vi "ACT_Loop.vi"() -> ()   [LabVIEW 2023, in "Angler_ACT.lvlib"]
uses:
  Angler_ACT.lvlib
  Cluster_CMD_ACT_Data.ctl
  ENUM_Input Mode.ctl
  Type Defs/Cluster_Angler_Angle to Position.ctl
  ENUM_ACT_State.ctl
  <vilib>/Rock Robotics/WPI/MotorControl/WPI_MotorControlDeviceRef.ctl
  <vilib>/Rock Robotics/WPI/MotorControl/WPI_MotorControlType.ctl
  <vilib>/Rock Robotics/SystemInterfaces/DIO/FPGA_DIOPWMChannel.ctl
  <vilib>/Rock Robotics/WPI/PWM/WPI_PWMDeadband.ctl
  <vilib>/Rock Robotics/SystemInterfaces/DIO/FPGA_DIOChannel.ctl
  <vilib>/Rock Robotics/WPI/ThirdParty/Phoenix-LabVIEW/Motor Controller/Controls/CTRE_Phoenix_MotorControl_NeutralMode.ctl
  <vilib>/Rock Robotics/WPI/ThirdParty/Phoenix-LabVIEW/Motor Controller/Controls/CTRE_Phoenix_MotorControl_ControlMode.ctl
  ENUM_ACT_Action.ctl
  RoboRIO Utilities/Global_STOP.vi
  Global_CMD_ACT_Data In.vi
  <vilib>/Rock Robotics/WPI/ThirdParty/Phoenix-LabVIEW/Motor Controller/Get/CTRE_Phoenix_MotorController_GetSelectedSensorData.vi
  <vilib>/Rock Robotics/WPI/ThirdParty/Phoenix-LabVIEW/Motor Controller/Get/CTRE_Phoenix_MotorController_GetClosedLoopData.vi
  Global_ACT_Data Out.vi
panel:
  in  "Max Speed":dbl=0.5
  out "Position Error":i32
  out "Current Angle":dbl
  in  "Angle vs Positon Table":T1[](array[typedef])=[{"Angle"=11.5, "Count"=100}, {"Angle"=15.0, "Count"=156}, {"Angle"=20.0, "Count"=231}, {"Angle"=25.0, "Count"=308}, {"Angle"=30.0, "Count"=386}, {"Angle"=35.0, "Count"=466}, {"Angle"=36.5, "Count"=480}]
  out "Target Unit Positon":dbl
  out "Input Angler Data":T2
  out "Sensor Positon":i32
  out "Cycle Time (S)":dbl format="%.3g"
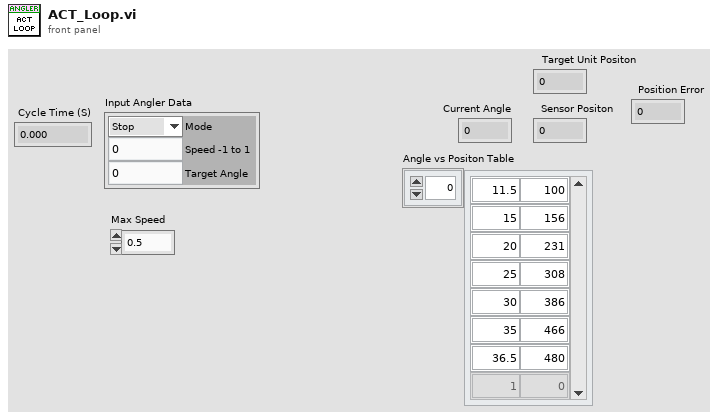
[diagram p1: front panel]
types:
  T1 = typedef "Cluster_Angler_Angle to Position.ctl" = cluster{"Angle":dbl, "Count":i32}
  T2 = typedef "Angler_ACT.lvlib/Cluster_CMD_ACT_Data.ctl" = cluster{"Mode":T3, "Speed -1 to 1":dbl, "Target Angle":dbl}
  T3 = typedef "Angler_ACT.lvlib/ENUM_Input Mode.ctl" = enum16{"Stop", "Speed", "Angle"}
  T4 = typedef "CTRE_Phoenix_MotorControl_ControlMode.ctl" = u16
  T5 = typedef "CTRE_Phoenix_MotorControl_NeutralMode.ctl" = enum8{"EEPROMSetting", "Override to Coast", "Override to Brake"}
  T6 = typedef "WPI_MotorControlDeviceRef.ctl" = cluster{"DeviceStatus":errorcluster, "Type":T7, "PWM":cluster{"PWM Channel":T8, "DeadBand":T9}, "CAN":cluster{"Device Number":u8, "SetOutput VI Ref":variant, "GetOutput VI Ref":variant, "Enable VI Ref":variant, "Disable VI Ref":variant, "Data":variant}, "Invert":bool, "DIO PWM":cluster{"PWM \"Enable\" Channel":T8, "DIOChannel":T10, "PWM Rate":dbl}}
  T7 = typedef "WPI_MotorControlType.ctl" = enum16{"PWM", "CAN", "DIO PWM"}
  T8 = typedef "FPGA_DIOPWMChannel.ctl" = enum8{"PWM 0", "PWM 1", "PWM 2", "PWM 3", "PWM 4", "PWM 5", "PWM 6", "PWM 7", "PWM 8", "PWM 9", "PWM MXP 0", "PWM MXP 1", "PWM MXP 2", "PWM MXP 3", "PWM MXP 4", "PWM MXP 5", "PWM MXP 6", "PWM MXP 7", "PWM MXP 8", "PWM MXP 9", "Invalid"}
  T9 = typedef "WPI_PWMDeadband.ctl" = cluster{"Name":string, "maxPositivePwm":i32, "minPositivePwm":i32, "centerPwm":i32, "maxNegativePwm":i32, "minNegativePwm":i32, "angularRange":u16}
  T10 = typedef "FPGA_DIOChannel.ctl" = enum8{"DIO 0", "DIO 1", "DIO 2", "DIO 3", "DIO 4", "DIO 5", "DIO 6", "DIO 7", "DIO 8", "DIO 9", "DIO MXP 0", "DIO MXP 1", "DIO MXP 2", "DIO MXP 3", "DIO MXP 4", "DIO MXP 5", "DIO MXP 6", "DIO MXP 7", "DIO MXP 8", "DIO MXP 9", "DIO MXP 10", "DIO MXP 11", "DIO MXP 12", "DIO MXP 13", "DIO MXP 14", "DIO MXP 15", "SPI Port CS1", "SPI Port CS2", "SPI Port CS3", "SPI Port MISO", "SPI Port MOSI", "Invalid"}
  T11 = typedef "Angler_ACT.lvlib/ENUM_ACT_State.ctl" = enum16{"Starting", "Stopping", "Ending", "Setting Speed", "Going to Angle"}
  T12 = typedef "Angler_ACT.lvlib/ENUM_ACT_Action.ctl" = enum16{"No Action", "Reset Time", "Reset All", "Stop", "Set Speed", "Set Target Position", "Calculate Target Position from Angle", "Set Soft Limits", "Set Min Motor Value", "Set Current Limit"}
  T13 = cluster{"Angler Motor Ref":T6, "State":T11, "Previous State":T11, "Current Time":timestamp, "Previous Time":timestamp, "Start Time":timestamp, "Target Time (ms)":u32, "Cycle Time(S)":dbl, "ACT Input":T2, "Target Unit Positon":dbl, "Current Angle":dbl, "Sensor Unit Position":i32, "Lower Soft Limit":bool, "Upper Soft Limit":bool, "Sensor Velocity":i32, "Control Mode":T4, "Motor Value":dbl, "Angle Array":dbl[], "Position Array":i32[], "Speed Limit":dbl, "Position Error":i32, "Min Motor Output":dbl, "Max Current":i32}
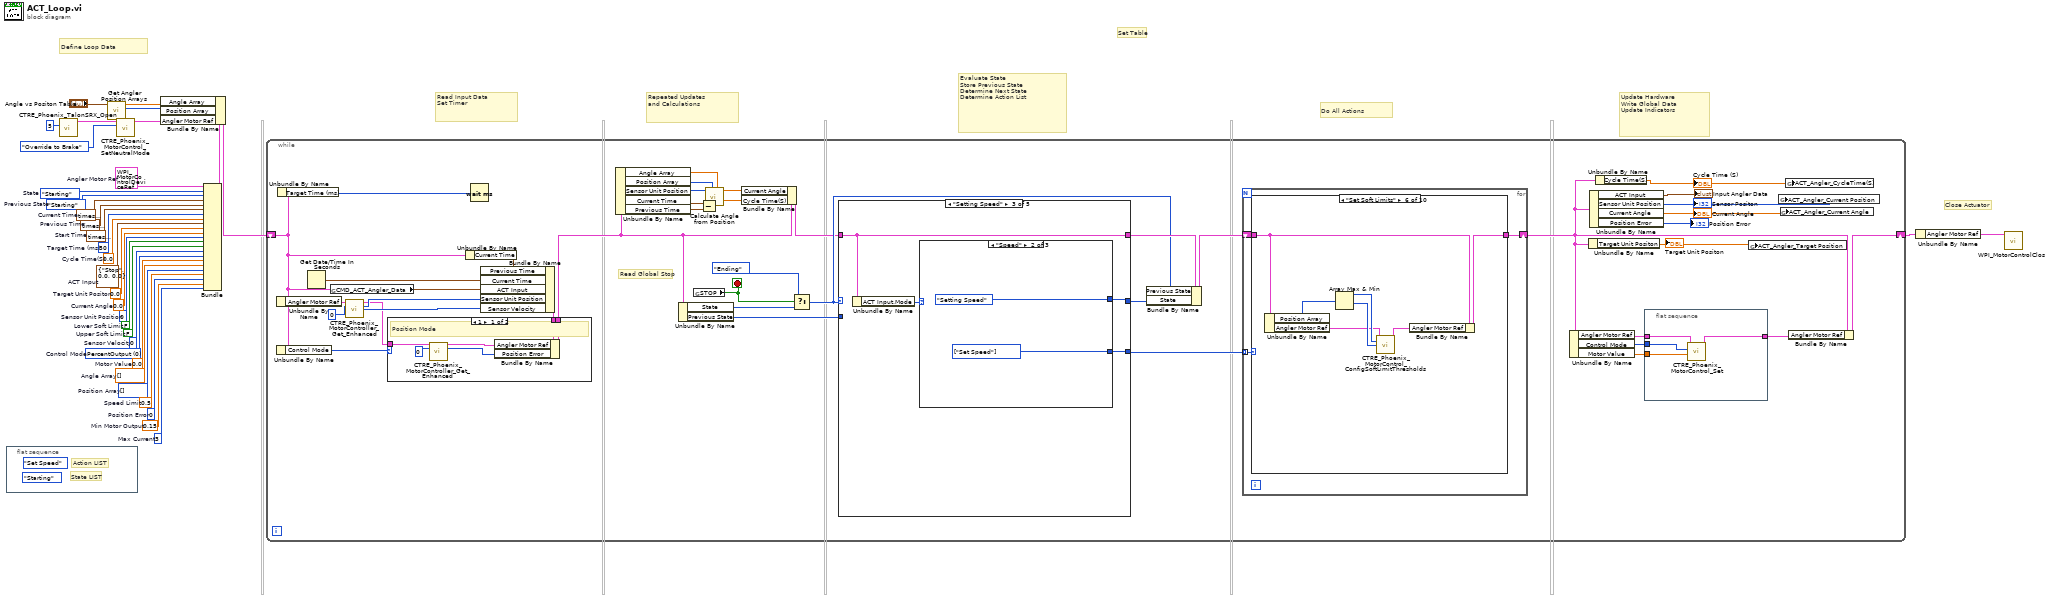
[diagram p0: block diagram]
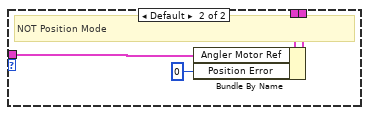
[diagram p2: hidden frame]
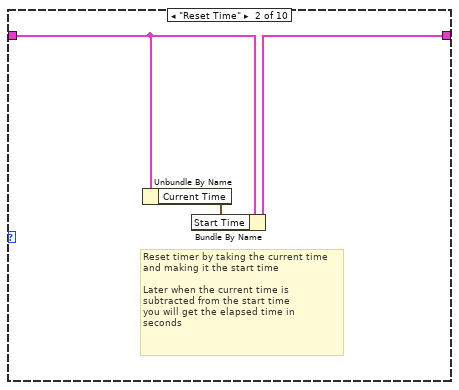
[diagram p4: hidden frame]
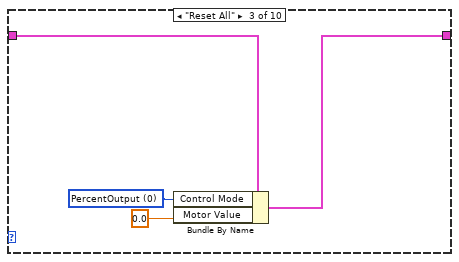
[diagram p5: hidden frame]
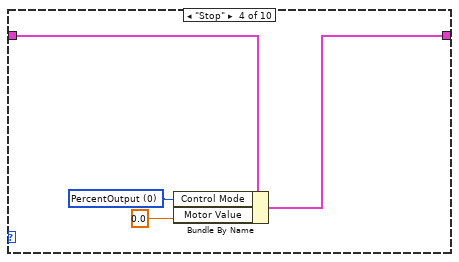
[diagram p6: hidden frame]
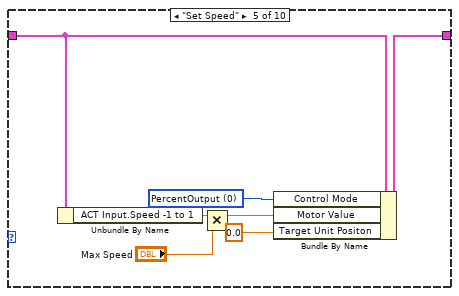
[diagram p7: hidden frame]
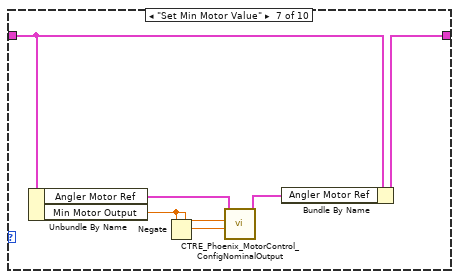
[diagram p8: hidden frame]
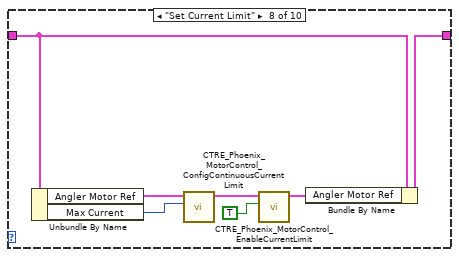
[diagram p9: hidden frame]
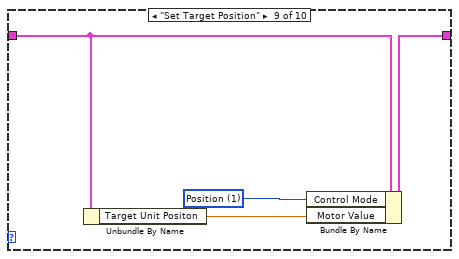
[diagram p10: hidden frame]
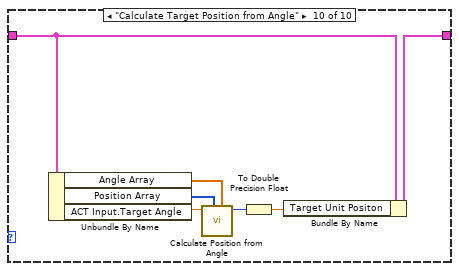
[diagram p11: hidden frame]
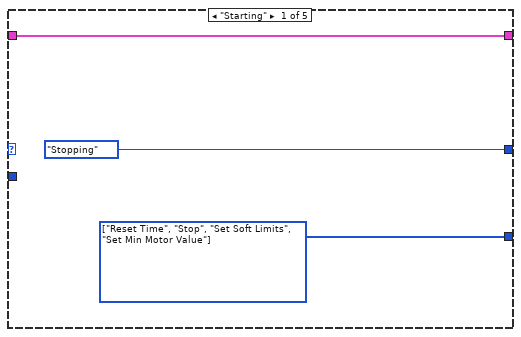
[diagram p12: hidden frame]
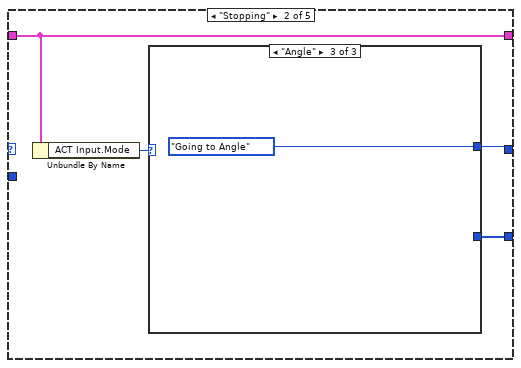
[diagram p13: hidden frame]
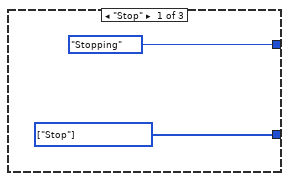
[diagram p14: hidden frame]
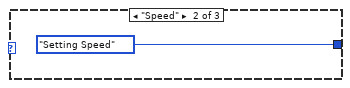
[diagram p15: hidden frame]
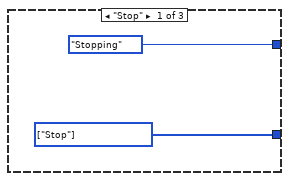
[diagram p16: hidden frame]
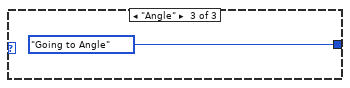
[diagram p17: hidden frame]
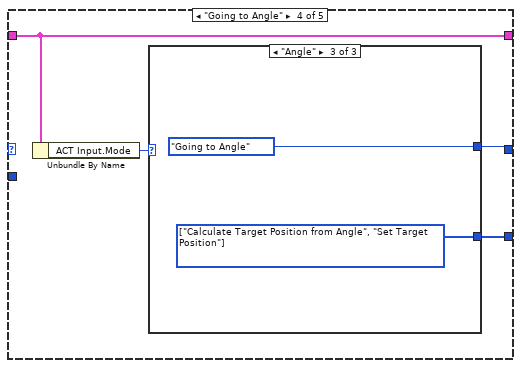
[diagram p18: hidden frame]
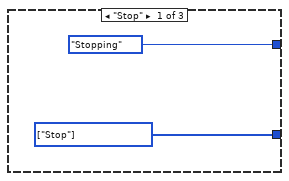
[diagram p19: hidden frame]
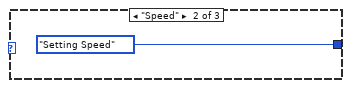
[diagram p20: hidden frame]
diagram:
  w1 = 3  # Max Current
  w2 = 0.15  # Min Motor Output
  w3 = 0  # Position Error
  w4 = 0.5  # Speed Limit
  w7 = i32[] []  # Position Array
  w8 = dbl[] []  # Angle Array
  w10 = 0.0  # Motor Value
  w11 = T4 0 items=["PercentOutput"=0, "Position"=1, "Velocity"=2, "Current"=3, "Follower"=5, "MotionProfile"=6, "MotionMagic"=7, "MotionProfileArc"=10, "Disabled"=15]  # Control Mode
  w12 = 0  # Sensor Velocity
  w16 = FALSE  # Upper Soft Limit
  w17 = FALSE  # Lower Soft Limit
  w18 = 0  # Sensor Unit Position
  w19 = 0.0  # Current Angle
  w22 = T6 {"DeviceStatus"={"status"=FALSE, "code"=0, "source"=""}, "Type"=enum."PWM", "PWM"={"PWM Channel"=enum."PWM 1", "DeadBand"={"Name"="", "maxPositivePwm"=0, "minPositivePwm"=0, "centerPwm"=0, "maxNegativePwm"=0, "minNegativePwm"=0, "angularRange"=0}}, "CAN"={"Device Number"=0, "SetOutput VI Ref"=variant(enum8{"Percent VBus", "Current", "Speed", "Position", "Voltage"} enum."Percent VBus"), "GetOutput VI Ref"=variant(refnum<k1> refnum), "Enable VI Ref"=variant(dbl 12.0), "Disable VI Ref"=variant(enum8{"Percent VBus", "Speed", "Position", "Slave", "Unchanged / Invalid", "Voltage Compensation", "Current", "Motion Profile"} enum."Percent VBus"), "Data"=variant}, "Invert"=FALSE, "DIO PWM"={"PWM \"Enable\" Channel"=enum."Invalid", "DIOChannel"=enum."Invalid", "PWM Rate"=0.0}}  # Angler Motor Ref
  w26 = 0.0  # Cycle Time(S)
  w27 = ENUM_ACT_State."Starting"  # Previous State
  w28 = timestamp(0 s since 1904-01-01)  # Previous Time
  w29 = u32 50  # Target Time (ms)
  w30 = 0.0  # Target Unit Positon
  w31 = T2 {"Mode"=enum."Stop", "Speed -1 to 1"=0.0, "Target Angle"=0.0}  # ACT Input
  w32 = timestamp(0 s since 1904-01-01)  # Start Time
  w33 = timestamp(0 s since 1904-01-01)  # Current Time
  w34 = ENUM_ACT_State."Starting"  # State
  # "Set Table"
  # "Close Actuator"
  # "Define Loop Data"
  # "Repeated Updates\nand Calculations"
  # "Read Input Data\nSet Timer"
  # "Evaluate State\nStore Previous State\nDetermine Next State\nDetermine Action List"
  # "Do All Actions"
  # "Update Hardware\nWrite Global Data\nUpdate Indicators"
  n1 = flat-sequence {
    frame #0 {
      (unwired) ENUM_ACT_State."Starting" ("State")
      (unwired) ENUM_ACT_Action."Set Speed" ("Action")
      # "State LIST"
      # "Action LIST"
    }
  }
  n2 = call <vilib>:"CTRE_Phoenix_TalonSRX_Open.vi"("Device Number"=u8 5) -> ("PhoenixMotorControlDevRef"=w14:T6)  [unwired: 9 in, 1 out]
  n3 = call "Get Angler Position Arrays.vi"("Position Array"="Angle vs Positon Table") -> ("Position Array"=w6:i32[], "Angle Array"=w5:dbl[])  [unwired: 9 in]
  n4 = call <vilib>:"CTRE_Phoenix_MotorControl_SetNeutralMode.vi"("Motor Control Neutral Mode"=CTRE_Phoenix_MotorControl_NeutralMode."Override to Brake", "PhoenixMotorControlDevRef"=w14) -> ("PhoenixMotorControlDevRef"=w13:T6)  [unwired: 8 in, 1 out]
  n5 = Bundle("Angler Motor Ref"=w22, "State"=w34, "Previous State"=w27, "Current Time"=w33, "Previous Time"=w28, "Start Time"=w32, "Target Time (ms)"=w29, "Cycle Time(S)"=w26, "ACT Input"=w31, "Target Unit Positon"=w30, "Current Angle"=w19, "Sensor Unit Position"=w18, "Lower Soft Limit"=w17, "Upper Soft Limit"=w16, "Sensor Velocity"=w12, "Control Mode"=w11, "Motor Value"=w10, "Angle Array"=w8, "Position Array"=w7, "Speed Limit"=w4, "Position Error"=w3, "Min Motor Output"=w2, "Max Current"=w1) -> (w24:T13)  [unwired: 1 in]
  n6 = Bundle By Name(cluster=w24, "Angle Array"=w5, "Position Array"=w6, "Angler Motor Ref"=w13) -> (w23:T13)
  n7 = while {
    shift-right: [w56] -> w25
    shift-left: w23 -> [w41]
    stop <- w72 stop-if-true
    # "Read Global Stop"
    n8 = Unbundle By Name(w41) -> ("Angler Motor Ref"=w52:T6)
    n9 = Unbundle By Name(w41) -> ("Control Mode"=w38:T4)
    n10 = Unbundle By Name(w41) -> ("Target Time (ms)"=w69:u32)
    n11 = Get Date/Time In Seconds() -> (seconds since 1Jan1904=w76:timestamp)
    n12 = global read "Global_CMD_ACT_Data In.vi" "CMD_ACT_Angler_Data"() -> (w59:T2)
    n13 = call-poly <vilib>:"CTRE_Phoenix_MotorController_Get_Enhanced.vi"("PhoenixMotorControlDevRef"=w52, "pidLoopIdx"=u32 0) -> ("PhoenixMotorControlDevRef"=w37:T6, "Position (Raw Sensor Units)"=w46:i32, "Velocity (Raw Sensor Units per 100 ms)"=w47:i32)  [unwired: 10 in, 1 out]
    n14 = Unbundle By Name(w41) -> ("Current Time"=w68:timestamp)
    n15 = Wait (ms)(milliseconds to wait=w69) -> ()  [unwired: 1 out]
    n16 = Bundle By Name(cluster=w41, "Previous Time"=w68, "Current Time"=w76, "ACT Input"=w59, "Sensor Unit Position"=w46, "Sensor Velocity"=w47) -> (w40:T13)
    n17 = case shown="1" w38 {
      tunnel: [w82 w86] -> w39
      tunnel: w40 -> [w81 w85]
      tunnel: w37 -> [w80 w84]
      frame 1 {
        # "Position Mode"
        n18 = call-poly <vilib>:"CTRE_Phoenix_MotorController_Get_Enhanced.vi"("PhoenixMotorControlDevRef"=w80, "pidLoopIdx"=0) -> ("PhoenixMotorControlDevRef"=w79:T6, "Closed-loop Error"=w78:i32)  [unwired: 8 in, 4 out]
        n19 = Bundle By Name(cluster=w81, "Angler Motor Ref"=w79, "Position Error"=w78) -> (w82:T13)
      }
      frame Default {
        # "NOT Position Mode"
        n20 = Bundle By Name(cluster=w85, "Angler Motor Ref"=w84, "Position Error"=0) -> (w86:T13)
      }
    }
    n21 = Unbundle By Name(w39) -> ("Angle Array"=w42:dbl[], "Position Array"=w43:i32[], "Sensor Unit Position"=w44:i32, "Current Time"=w64:timestamp, "Previous Time"=w65:timestamp)
    n22 = Unbundle By Name(w39) -> ("State"=w70:T11, "Previous State"=w67:T11)
    n23 = global read "Global_STOP.vi" "STOP"() -> (w72:bool)
    n24 = Subtract(x=w64, y=w65) -> (x-y=w62:dbl)
    n25 = call "Calculate Angle from Position.vi"("Angle Array"=w42, "Position Array"=w43, "Sensor Unit Position"=w44) -> ("Current Angle"=w45:dbl)  [unwired: 8 in]
    n26 = Bundle By Name(cluster=w39, "Current Angle"=w45, "Cycle Time(S)"=w62) -> (w63:T13)
    n27 = Select(t=ENUM_ACT_State."Ending" ("State"), s=w72, f=w70) -> (s? t:f=w66:T11)
    n28 = case shown="\"Setting Speed\"" w66 {
      tunnel: w63 -> [w146 w150 w158 w167 w175]
      tunnel: [w146 w150 w158 w167 w175] -> w74
      tunnel: [ENUM_ACT_State."Stopping" ("State") w148 w156 w165 ENUM_ACT_State."Ending" ("State")] -> w73
      tunnel: [w145 w147 w155 w164 w173] -> w61
      tunnel: w67 -> [_ _ _ _ _]
      frame "Starting" {
        w145 = T12[] [enum."Reset Time", enum."Stop", enum."Set Soft Limits", enum."Set Min Motor Value"] items=["No Action", "Reset Time", "Reset All", "Stop", "Set Speed", "Set Target Position", "Calculate Target Position from Angle", "Set Soft Limits", "Set Min Motor Value", "Set Current Limit"] ("Actions")
      }
      frame "Stopping" {
        n29 = Unbundle By Name(w150) -> ("ACT Input.Mode"=w149:T3)
        n30 = case shown="\"Angle\"" w149 {
          tunnel: [ENUM_ACT_State."Stopping" ("State") ENUM_ACT_State."Setting Speed" ("State") ENUM_ACT_State."Going to Angle" ("State")] -> w148
          tunnel: [w151 _ _] -> w147
          frame "Stop" {
            w151 = T12[] [enum."Stop"] items=["No Action", "Reset Time", "Reset All", "Stop", "Set Speed", "Set Target Position", "Calculate Target Position from Angle", "Set Soft Limits", "Set Min Motor Value", "Set Current Limit"] ("Actions")
          }
          frame "Speed" {
          }
          frame "Angle" {
          }
        }
      }
      frame "Setting Speed" {
        n31 = Unbundle By Name(w158) -> ("ACT Input.Mode"=w157:T3)
        n32 = case shown="\"Speed\"" w157 {
          tunnel: [ENUM_ACT_State."Stopping" ("State") ENUM_ACT_State."Setting Speed" ("State") ENUM_ACT_State."Going to Angle" ("State")] -> w156
          tunnel: [w159 w161 _] -> w155
          frame "Stop" {
            w159 = T12[] [enum."Stop"] items=["No Action", "Reset Time", "Reset All", "Stop", "Set Speed", "Set Target Position", "Calculate Target Position from Angle", "Set Soft Limits", "Set Min Motor Value", "Set Current Limit"] ("Actions")
          }
          frame "Speed" {
            w161 = T12[] [enum."Set Speed"] items=["No Action", "Reset Time", "Reset All", "Stop", "Set Speed", "Set Target Position", "Calculate Target Position from Angle", "Set Soft Limits", "Set Min Motor Value", "Set Current Limit"] ("Actions")
          }
          frame "Angle" {
          }
        }
      }
      frame "Going to Angle" {
        n33 = Unbundle By Name(w167) -> ("ACT Input.Mode"=w166:T3)
        n34 = case shown="\"Angle\"" w166 {
          tunnel: [ENUM_ACT_State."Stopping" ("State") ENUM_ACT_State."Setting Speed" ("State") ENUM_ACT_State."Going to Angle" ("State")] -> w165
          tunnel: [w168 _ w171] -> w164
          frame "Stop" {
            w168 = T12[] [enum."Stop"] items=["No Action", "Reset Time", "Reset All", "Stop", "Set Speed", "Set Target Position", "Calculate Target Position from Angle", "Set Soft Limits", "Set Min Motor Value", "Set Current Limit"] ("Actions")
          }
          frame "Speed" {
          }
          frame "Angle" {
            w171 = T12[] [enum."Calculate Target Position from Angle", enum."Set Target Position"] items=["No Action", "Reset Time", "Reset All", "Stop", "Set Speed", "Set Target Position", "Calculate Target Position from Angle", "Set Soft Limits", "Set Min Motor Value", "Set Current Limit"] ("Actions")
          }
        }
      }
      frame "Ending" {
        w173 = T12[] [enum."Reset All"] items=["No Action", "Reset Time", "Reset All", "Stop", "Set Speed", "Set Target Position", "Calculate Target Position from Angle", "Set Soft Limits", "Set Min Motor Value", "Set Current Limit"] ("Actions")
      }
    }
    n35 = Bundle By Name(cluster=w74, "Previous State"=w66, "State"=w73) -> (w75:T13)
    n36 = for {
      tunnel: w61 -> [w93] mode=indexing
      shift-right: [w92] -> w49
      shift-left: w75 -> [w91]
      n37 = case shown="\"Set Soft Limits\"" w93 {
        tunnel: w91 -> [w94 w97 w101 w105 w110 w118 w124 w131 w134 w142]
        tunnel: [w94 w96 w100 w104 w112 w119 w125 w132 w136 w143] -> w92
        frame "No Action" {
        }
        frame "Reset Time" {
          # "Reset timer by taking the current time\nand making it the start time\n\nLater when the current time is \nsubtracted from the start time\nyou will get the elapsed time in \nseconds"
          n38 = Unbundle By Name(w97) -> ("Current Time"=w95:timestamp)
          n39 = Bundle By Name(cluster=w97, "Start Time"=w95) -> (w96:T13)
        }
        frame "Reset All" {
          w99 = T4 0 items=["PercentOutput"=0, "Position"=1, "Velocity"=2, "Current"=3, "Follower"=5, "MotionProfile"=6, "MotionMagic"=7, "MotionProfileArc"=10, "Disabled"=15] ("Control Mode")
          n40 = Bundle By Name(cluster=w101, "Control Mode"=w99, "Motor Value"=0.0) -> (w100:T13)
        }
        frame "Stop" {
          w103 = T4 0 items=["PercentOutput"=0, "Position"=1, "Velocity"=2, "Current"=3, "Follower"=5, "MotionProfile"=6, "MotionMagic"=7, "MotionProfileArc"=10, "Disabled"=15] ("Control Mode")
          n41 = Bundle By Name(cluster=w105, "Control Mode"=w103, "Motor Value"=0.0) -> (w104:T13)
        }
        frame "Set Speed" {
          w111 = T4 0 items=["PercentOutput"=0, "Position"=1, "Velocity"=2, "Current"=3, "Follower"=5, "MotionProfile"=6, "MotionMagic"=7, "MotionProfileArc"=10, "Disabled"=15] ("Control Mode")
          n42 = Unbundle By Name(w110) -> ("ACT Input.Speed -1 to 1"=w109:dbl)
          n43 = Multiply(x=w109, y="Max Speed") -> (x*y=w107:dbl)
          n44 = Bundle By Name(cluster=w110, "Control Mode"=w111, "Motor Value"=w107, "Target Unit Positon"=0.0) -> (w112:T13)
        }
        frame "Set Soft Limits" {
          n45 = Unbundle By Name(w118) -> ("Position Array"=w117:i32[], "Angler Motor Ref"=w114:T6)
          n46 = Array Max & Min(array=w117) -> (max value=w116:i32, min value=w115:i32)  [unwired: 2 out]
          n47 = call <vilib>:"CTRE_Phoenix_MotorControl_ConfigSoftLimitThresholds.vi"("PhoenixMotorControlDevRef"=w114, "Forward Soft Limit"=w116, "Reverse Soft Limit"=w115) -> ("PhoenixMotorControlDevRef"=w113:T6)  [unwired: 11 in, 1 out]
          n48 = Bundle By Name(cluster=w118, "Angler Motor Ref"=w113) -> (w119:T13)
        }
        frame "Set Min Motor Value" {
          n49 = Unbundle By Name(w124) -> ("Angler Motor Ref"=w123:T6, "Min Motor Output"=w121:dbl)
          n50 = Negate(x=w121) -> (-x=w120:dbl)
          n51 = call <vilib>:"CTRE_Phoenix_MotorControl_ConfigNominalOutput.vi"("Reverse Nominal Percent Output"=w120, "Forward Nominal Percent Output"=w121, "PhoenixMotorControlDevRef"=w123) -> ("PhoenixMotorControlDevRef"=w122:T6)  [unwired: 7 in, 1 out]
          n52 = Bundle By Name(cluster=w124, "Angler Motor Ref"=w122) -> (w125:T13)
        }
        frame "Set Current Limit" {
          n53 = Unbundle By Name(w131) -> ("Angler Motor Ref"=w130:T6, "Max Current"=w129:i32)
          n54 = call <vilib>:"CTRE_Phoenix_MotorControl_ConfigContinuousCurrentLimit.vi"("Continuous Current Limit (Amps)"=w129, "PhoenixMotorControlDevRef"=w130) -> ("PhoenixMotorControlDevRef"=w128:T6)  [unwired: 8 in, 1 out]
          n55 = call <vilib>:"CTRE_Phoenix_MotorControl_EnableCurrentLimit.vi"("Enable Current Limit?"=TRUE, "PhoenixMotorControlDevRef"=w128) -> ("PhoenixMotorControlDevRef"=w127:T6)  [unwired: 8 in, 1 out]
          n56 = Bundle By Name(cluster=w131, "Angler Motor Ref"=w127) -> (w132:T13)
        }
        frame "Set Target Position" {
          w135 = T4 1 items=["PercentOutput"=0, "Position"=1, "Velocity"=2, "Current"=3, "Follower"=5, "MotionProfile"=6, "MotionMagic"=7, "MotionProfileArc"=10, "Disabled"=15] ("Control Mode")
          n57 = Unbundle By Name(w134) -> ("Target Unit Positon"=w133:dbl)
          n58 = Bundle By Name(cluster=w134, "Control Mode"=w135, "Motor Value"=w133) -> (w136:T13)
        }
        frame "Calculate Target Position from Angle" {
          n59 = Unbundle By Name(w142) -> ("Angle Array"=w137:dbl[], "Position Array"=w138:i32[], "ACT Input.Target Angle"=w141:dbl)
          n60 = call "Calculate Position from Angle.vi"("Angle Array"=w137, "Position Array"=w138, "Angle"=w141) -> ("Sensor Unit Position Out"=w140:i32)  [unwired: 8 in]
          n61 = To Double Precision Float(number=w140) -> (double precision float=w139:dbl)
          n62 = Bundle By Name(cluster=w142, "Target Unit Positon"=w139) -> (w143:T13)
        }
      }
    }
    n63 = Unbundle By Name(w49) -> ("Angler Motor Ref"=w58:T6, "Control Mode"=w54:T4, "Motor Value"=w53:dbl)
    n64 = Unbundle By Name(w49) -> ("Target Unit Positon"=w48:dbl)
    "Target Unit Positon" <- w48
    n65 = Unbundle By Name(w49) -> ("ACT Input"=→"Input Angler Data":T2, "Sensor Unit Position"=w36:i32, "Current Angle"=w50:dbl, "Position Error"=→"Position Error":i32)
    "Sensor Positon" <- w36
    "Current Angle" <- w50
    n66 = Unbundle By Name(w49) -> ("Cycle Time(S)"=w55:dbl)
    "Cycle Time (S)" <- w55
    n67 = flat-sequence {
      tunnel: w58 -> [w89]
      tunnel: [w90] -> w57
      tunnel: w54 -> [w88]
      tunnel: w53 -> [w87]
      frame #0 {
        n68 = call <vilib>:"CTRE_Phoenix_MotorControl_Set.vi"("Output"=w87, "Control Mode"=w88, "PhoenixMotorControlDevRef"=w89) -> ("PhoenixMotorControlDevRef"=w90:T6)  [unwired: 7 in, 1 out]
      }
    }
    n69 = global write "Global_ACT_Data Out.vi" "ACT_Angler_Target Position"(w48) -> ()
    n70 = global write "Global_ACT_Data Out.vi" "ACT_Angler_Current Position"(w36) -> ()
    n71 = global write "Global_ACT_Data Out.vi" "ACT_Angler_Current Angle"(w50) -> ()
    n72 = global write "Global_ACT_Data Out.vi" "ACT_Angler_CycleTime(S)"(w55) -> ()
    n73 = Bundle By Name(cluster=w49, "Angler Motor Ref"=w57) -> (w56:T13)
  }
  n74 = Unbundle By Name(w25) -> ("Angler Motor Ref"=w20:T6)
  n75 = call <vilib>:"WPI_MotorControlClose.vi"("MotorControlDevRef"=w20) -> ()  [unwired: 10 in, 1 out]
